vi "instr.FunctionGenerator.vi"(7 "Model":enum16{"UEL20D", "ATF20D+"}(ring), 8 "error in (no error)":errorcluster caption="错误输入（无错误）", 9 "Vpp(mVpp)":u32, 10 "Freq(Hz)":u64, 11 "VISA resource name":refnum<visa-resource-name>="COM1" caption="RS232") -> (0 "error out":errorcluster caption="错误输出", 3 "OK?":bool)   [LabVIEW 2012, in "Lib_UEL.ATE.lvlib" / "Lib_Instrument.lvlib"]
uses:
  Lib_Instrument.lvlib
panel:
  in  "CMD":enum16{"SET_Signal", "SET_Close", "CHK_Status"}(ring)
  in  "timeout (10sec)":u32=1000 caption="超时（10秒）"
  # "2012-12-06: Initial version.\n旧版本,使用字节命令来操作旧版DDS.\n新版DDS使用SCPI命令操作, 本VI旧功能已废弃.\n----------------------\nV1.0.0 2015-7-8\nDDS FG API, 兼容ATF20D+和UEL20D."
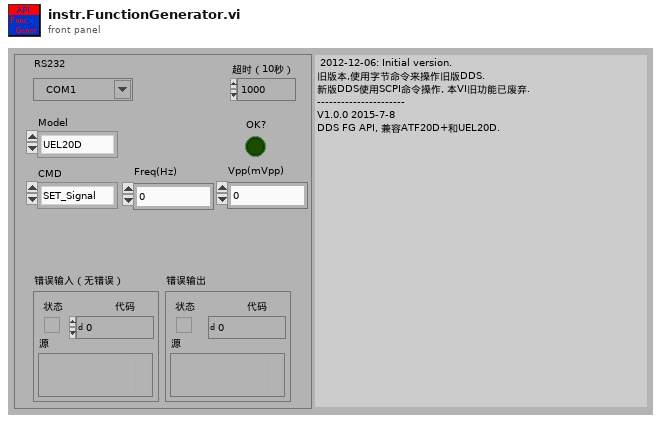
[diagram p1: front panel]
types:
  T1 = enum16{"MHz", "kHz", "Hz", "Vpp", "mVpp", "Vrms", "mVrms", "No."}
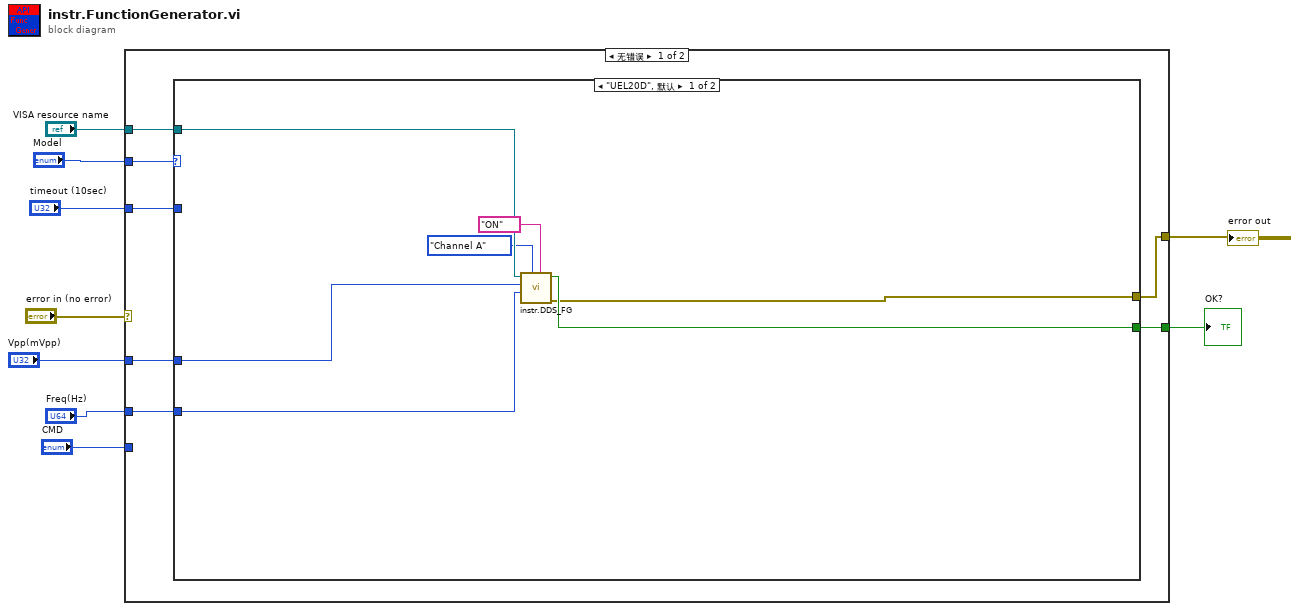
[diagram p0: block diagram]
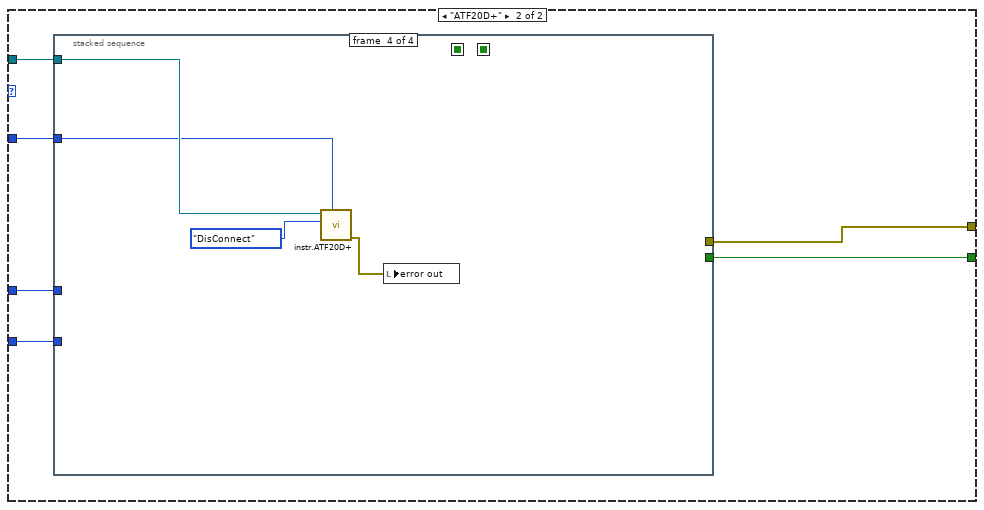
[diagram p2: hidden frame]
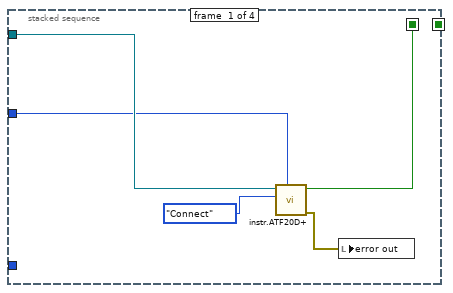
[diagram p3: hidden frame]
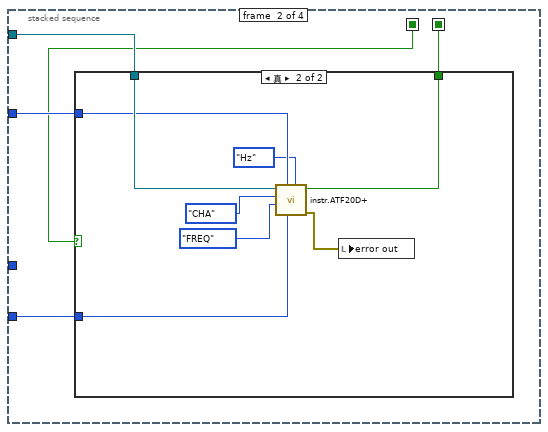
[diagram p4: hidden frame]
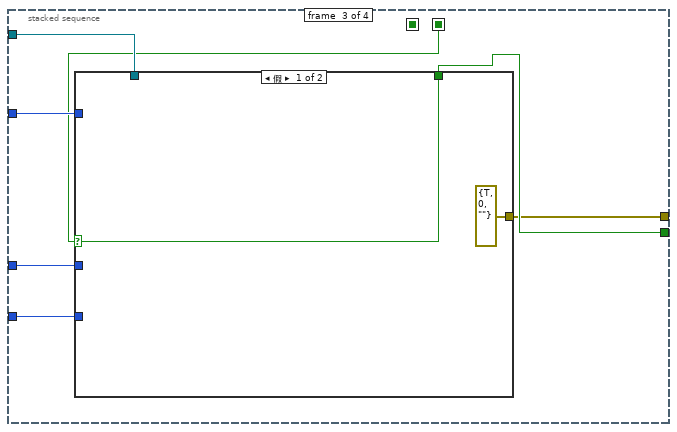
[diagram p6: hidden frame]
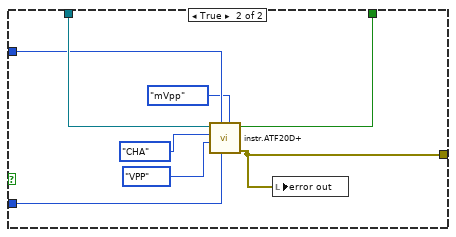
[diagram p7: hidden frame]
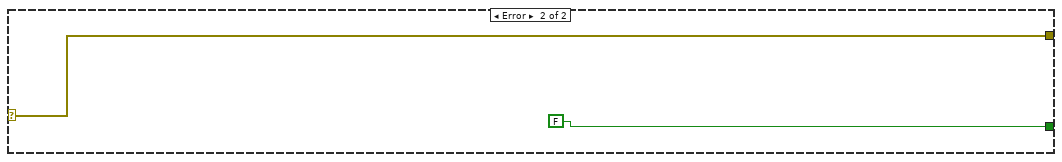
[diagram p8: hidden frame]
diagram:
  n1 = case shown="无错误" "error in (no error)" {
    selector: "error in (no error)" -> [_ w71]
    tunnel: "VISA resource name" -> [w15 _]
    tunnel: [w10 w71] -> w6
    tunnel: "timeout (10sec)" -> [w14 _]
    tunnel: "Freq(Hz)" -> [w13 _]
    tunnel: "CMD" -> [_ _]
    tunnel: "Model" -> [w16 _]
    tunnel: [w12 FALSE ("OK?")] -> w2
    tunnel: "Vpp(mVpp)" -> [w11 _]
    frame No Error {
      n2 = case shown="\"UEL20D\", 默认" w16 {
        tunnel: w15 -> [w23 w29]
        tunnel: w14 -> [_ w28]
        tunnel: w13 -> [w21 w27]
        tunnel: [w18 w26] -> w12
        tunnel: w11 -> [w22 w25]
        tunnel: [w17 w24] -> w10
        frame "UEL20D", Default {
          n3 = call "instr.DDS_FG.vi"("SWITCH"="ON", "CH"=enum16{"Channel A", "Channel B", "Both"}."Channel A", "FREQ"=w21, "AMP"=w22, "COM"=w23) -> ("Error Out"=w17:errorcluster, "STA"=w18:bool)  [unwired: 5 in]
        }
        frame "ATF20D+" {
          n4 = stacked-sequence {
            seq-local: [w30 _ _ _] -> [_ w37 _ _]
            seq-local: [_ w35 _ _] -> [_ _ w52 _]
            tunnel: w29 -> [w34 w39 w55 w69]
            tunnel: w28 -> [w33 w38 w54 w68]
            tunnel: w27 -> [_ w36 w53 _]
            tunnel: [_ _ w51 _] -> w26
            tunnel: w25 -> [_ _ w50 _]
            tunnel: [_ _ w49 _] -> w24
            frame #0 {
              n5 = call "instr.ATF20D+.vi"("timeout (10sec)"=w33, "Channel"=enum16{"CHA", "CHB", "Connect", "DisConnect"}."Connect", "VISA resource name"=w34) -> ("error out"=w31:errorcluster, "OK?"=w30:bool)  [unwired: 4 in, 3 out]
              n6 = local write "error out"(w31) -> ()
            }
            frame #1 {
              n7 = case shown="真" w37 {
                selector: w37 -> [w40 _]
                tunnel: w39 -> [_ w48]
                tunnel: w38 -> [_ w47]
                tunnel: w36 -> [_ w42]
                tunnel: [w40 w41] -> w35
                frame False {
                }
                frame True {
                  n8 = call "instr.ATF20D+.vi"("Unit"=T1."Hz", "Para"=w42, "timeout (10sec)"=w47, "CMD"=enum16{"FREQ", "VPP", "VRMS", "SWITCH"}."FREQ", "Channel"=enum16{"CHA", "CHB", "Connect", "DisConnect"}."CHA", "VISA resource name"=w48) -> ("error out"=w45:errorcluster, "OK?"=w41:bool)  [unwired: 1 in, 3 out]
                  n9 = local write "error out"(w45) -> ()
                }
              }
            }
            frame #2 {
              n10 = case shown="假" w52 {
                selector: w52 -> [w57 _]
                tunnel: w55 -> [_ w65]
                tunnel: w54 -> [_ w64]
                tunnel: w53 -> [_ _]
                tunnel: [w57 w60] -> w51
                tunnel: w50 -> [_ w59]
                tunnel: [errorcluster {"status"=TRUE, "code"=0, "source"=""} ("error out") w58] -> w49
                frame False {
                }
                frame True {
                  n11 = call "instr.ATF20D+.vi"("Unit"=T1."mVpp", "Para"=w59, "timeout (10sec)"=w64, "CMD"=enum16{"FREQ", "VPP", "VRMS", "SWITCH"}."VPP", "Channel"=enum16{"CHA", "CHB", "Connect", "DisConnect"}."CHA", "VISA resource name"=w65) -> ("error out"=w58:errorcluster, "OK?"=w60:bool)  [unwired: 1 in, 3 out]
                  n12 = local write "error out"(w58) -> ()
                }
              }
            }
            frame #3 {
              n13 = call "instr.ATF20D+.vi"("timeout (10sec)"=w68, "Channel"=enum16{"CHA", "CHB", "Connect", "DisConnect"}."DisConnect", "VISA resource name"=w69) -> ("error out"=w66:errorcluster)  [unwired: 4 in, 4 out]
              n14 = local write "error out"(w66) -> ()
            }
          }
        }
      }
    }
    frame Error {
    }
  }
  "error out" <- w6
  "OK?" <- w2
